vi "TDT-Get Events Final.vi"(0 "Data":T1={"TTankX"=refnum, "TDevAccX"=refnum, "LastTime"=0.0, "error"={"status"=FALSE, "code"=0, "source"=""}, "Block Name"="", "Circuit Tag"="", "Tank Name"="", "NumTicks"=0, "LastTick"=0.0, "Idle?"=FALSE, "Wait (ms)"=1000, "LastArtf"=0.0, "LastTosc"=0.0}, 11 "error in (no error)":errorcluster, 13 "Tetrode":bool) -> (4 "Data out":T1={"TTankX"=refnum, "TDevAccX"=refnum, "LastTime"=0.0, "error"={"status"=FALSE, "code"=0, "source"=""}, "Block Name"="", "Circuit Tag"="", "Tank Name"="", "NumTicks"=0, "LastTick"=0.0, "Idle?"=FALSE, "Wait (ms)"=1000, "LastArtf"=0.0, "LastTosc"=0.0}, 8 "Events":dbl[][](array[numeric]), 10 "total ticks":i32, 15 "error out":errorcluster)   [LabVIEW 2015]
uses:
  TDT Interface Data.ctl
panel:
  out "NumTicks":i32
  in  "Poll Interval (s)":dbl=2.0
  in  "Timeout (s)":dbl=10.0
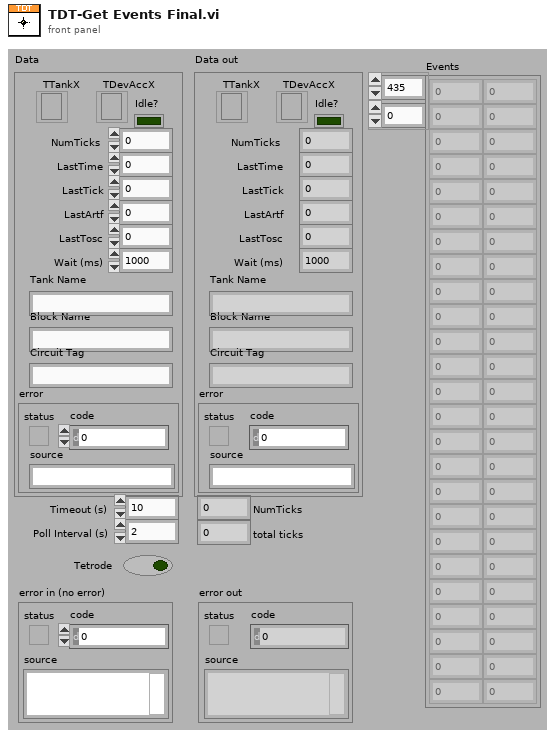
[diagram p1: front panel]
types:
  T1 = typedef "TDT Interface Data.ctl" = cluster{"TTankX":refnum<k7>, "TDevAccX":refnum<k7>, "LastTime":dbl, "error":errorcluster, "Block Name":string, "Circuit Tag":string, "Tank Name":string, "NumTicks":i32, "LastTick":dbl, "Idle?":bool, "Wait (ms)":u32, "LastArtf":dbl, "LastTosc":dbl}
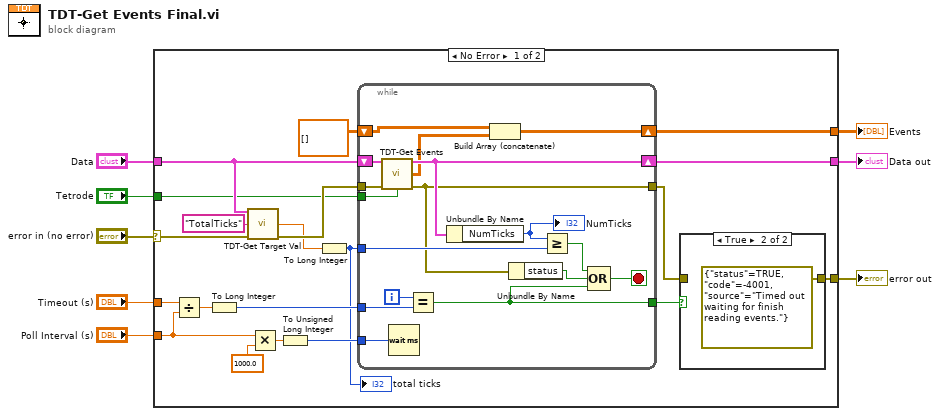
[diagram p0: block diagram]
diagram:
  n1 = case shown="No Error" "error in (no error)" {
    selector: "error in (no error)" -> [w14 w49]
    tunnel: [w20 w49] -> w7
    tunnel: "Data" -> [w11 w48]
    tunnel: "Timeout (s)" -> [w25 _]
    tunnel: "Poll Interval (s)" -> [w24 _]
    tunnel: [w17 w48] -> w3
    tunnel: [w16 _] -> w2
    tunnel: "Tetrode" -> [w9 _]
    frame No Error {
      n2 = Divide(x=w25, y=w24) -> (x/y=w28:dbl)
      n3 = To Long Integer(number=w28) -> (32bit integer=w22:i32)
      n4 = call "TDT-Get Target Val.vi"("Data"=w11, "Target"="TotalTicks", "error in (no error)"=w14) -> ("GetTargetVal"=w12:dbl, "error out"=w13:errorcluster)  [unwired: 11 in]
      n5 = Multiply(x=w24, y=1000.0) -> (x*y=w27:dbl)
      n6 = To Unsigned Long Integer(number=w27) -> (unsigned 32bit integer=w23:u32)
      n7 = To Long Integer(number=w12) -> (32bit integer=w19:i32)
      "total ticks" <- w19
      n8 = while {
        tunnel: w13 -> [w40]
        tunnel: w23 -> [w46]
        tunnel: w22 -> [w44]
        tunnel: [w42] -> w21
        tunnel: w19 -> [w37]
        shift-right: [w39] -> w17
        shift-left: w11 -> [w41]
        tunnel: [w35] -> w18
        shift-right: [w33] -> w16
        shift-left: dbl[][] [] -> [w32]
        tunnel: w9 -> [w31]
        i -> [w45]
        stop <- w47 stop-if-true
        n9 = call "TDT-Get Events.vi"("Data"=w41, "error in (no error)"=w40, "Tetrode"=w31) -> ("Data out"=w39:T1, "Events"=w34:dbl[][], "error out"=w35:errorcluster)  [unwired: 10 in]
        n10 = Wait (ms)(milliseconds to wait=w46) -> ()  [unwired: 1 out]
        n11 = Equal?(x=w45, y=w44) -> (x = y?=w42:bool)
        n12 = Unbundle By Name(w39) -> ("NumTicks"=w38:i32)
        "NumTicks" <- w38
        n13 = Build Array (concatenate)(w32, w34) -> (w33:dbl[][])
        n14 = Unbundle By Name(w35) -> ("status"=w36:bool)
        n15 = Greater Or Equal?(x=w38, y=w37) -> (x >= y?=w43:bool)
        n16 = Compound Arithmetic op=OR(w43, w36, w42) -> (w47:bool)
      }
      n17 = case shown="True" w21 {
        tunnel: [w29 errorcluster {"status"=TRUE, "code"=-4001, "source"="Timed out waiting for finish reading events."} ("error out")] -> w20
        tunnel: w18 -> [w29 _]
        frame False {
        }
        frame True {
        }
      }
    }
    frame Error {
    }
  }
  "error out" <- w7
  "Data out" <- w3
  "Events" <- w2
